vi "task_manager.vi"(8 "error out 2":errorcluster) -> (0 "error out":errorcluster)   [LabVIEW 2010]
uses:
  <userlib>/_OpenG.lib/array/array.llb/Sort 1D Array (String)__ogtk.vi
  <userlib>/_OpenG.lib/array/array.llb/Sort 2D Array (String)__ogtk.vi
panel:
  in  "sort by":u32(ring) items=["Name", "Type", "State", "Size", "Clones"]
  in  "stop":bool
  in  "end process":bool
  in  "VIs in Memory:":i32(listbox)
  # "Task Manager"
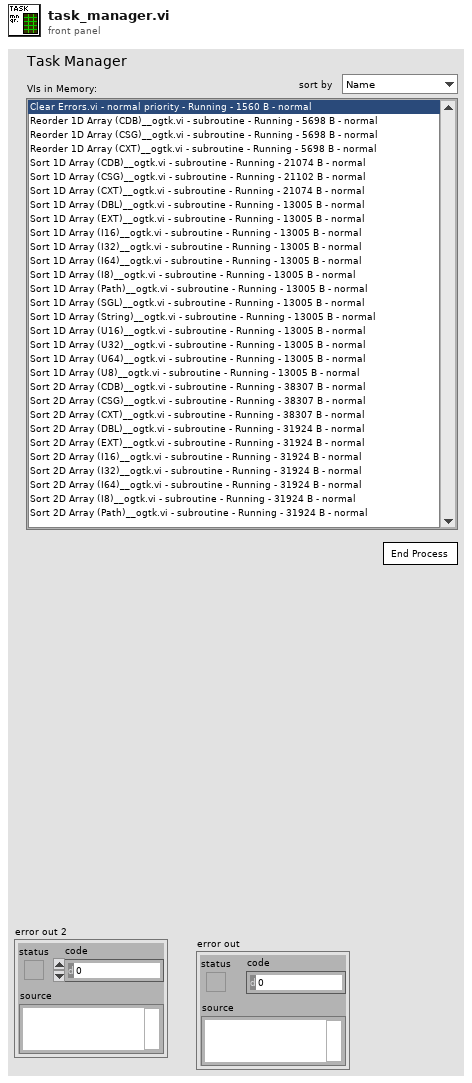
[diagram p1: front panel]
types:
  T1 = enum32{"invalid priority", "background priority", "normal priority", "above normal priority", "high priority", "time critical priority", "subroutine"}
  T2 = enum32{"Bad", "Idle", "Run top level", "Running"}
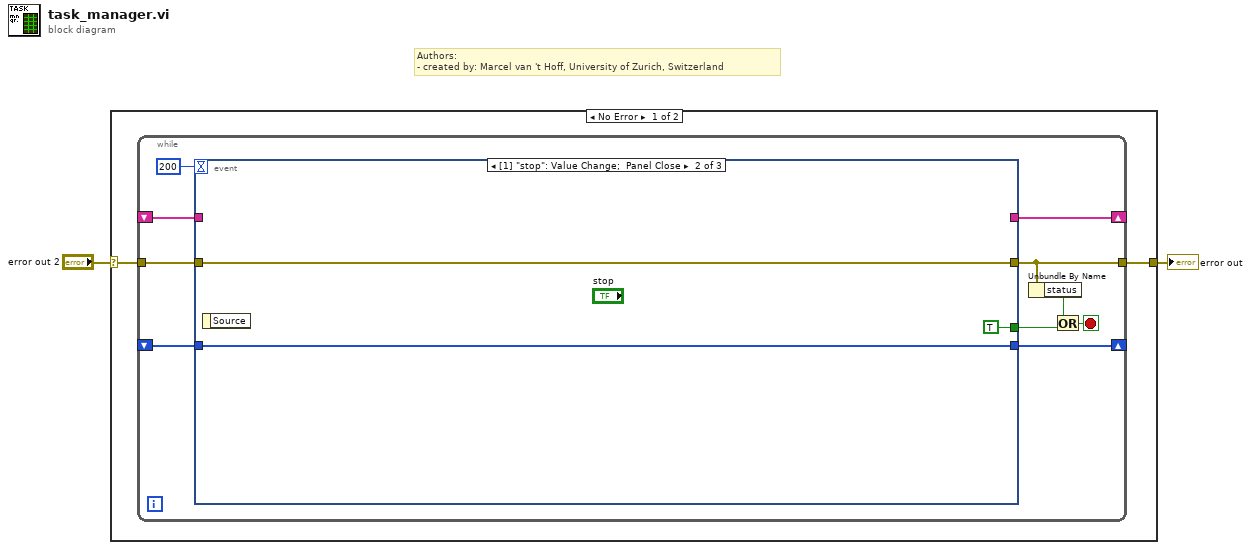
[diagram p0: block diagram]
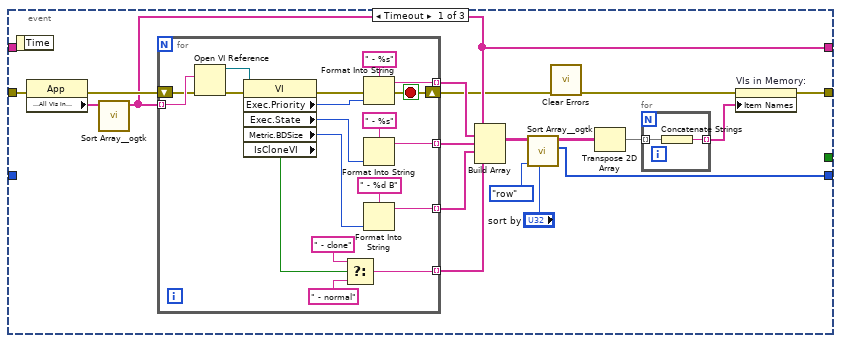
[diagram p2: hidden frame]
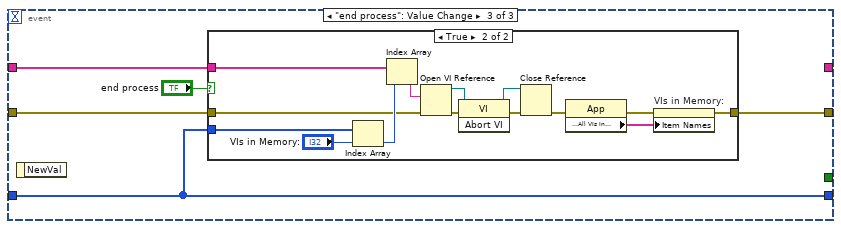
[diagram p3: hidden frame]
diagram:
  # "Authors: \n- created by: Marcel van 't Hoff, University of Zurich, Switzerland"
  n1 = case shown="No Error" "error out 2" {
    selector: "error out 2" -> [w3 w77]
    tunnel: [w4 w77] -> w2
    frame No Error {
      n2 = while {
        shift-right: [w13] -> _
        shift-left: _ -> [w12]
        shift-right: [w11] -> _
        shift-left: _ -> [w10]
        tunnel: [w8] -> w4
        tunnel: w3 -> [w9]
        stop <- w5 stop-if-true
        n3 = event shown="[1] \"stop\": Value Change;  Panel Close" {
          selector: _ -> [_ _ _]
          dyn-events: _ -> [_ _ _]
          timeout: 200 -> [_ _ _]
          tunnel: [_ TRUE ("stop") _] -> w6
          tunnel: [w18 _ _] -> w13
          tunnel: w12 -> [_ _ w60]
          tunnel: [w22 w56 w59] -> w11
          tunnel: w10 -> [_ w56 w59]
          tunnel: [w20 w55 w58] -> w8
          tunnel: w9 -> [w21 w55 w57]
          event Timeout {
            n4 = event-data() -> ()  [unwired: 1 in, 1 out]
            n5 = property class="App"(error in=w21) -> (error out=w19:errorcluster, "Application:All VIs In Memory"=w23:string[])  [unwired: 1 in, 1 out]
            n6 = call-poly <userlib>:"Sort Array__ogtk.vi"("Array in"=w23) -> ("Sorted Array out"=w18:string[])  [unwired: 9 in, 1 out]
            n7 = for {
              tunnel: w18 -> [w52] mode=indexing
              tunnel: [w46] -> w32 mode=indexing
              tunnel: [w45] -> w30 mode=indexing
              tunnel: [w44] -> w29 mode=indexing
              shift-right: [w39] -> w17
              shift-left: w19 -> [w41]
              tunnel: [w37] -> w16 mode=indexing
              stop <- w39 stop-if-true
              n8 = Open VI Reference(vi path=w52, error in (no error)=w41) -> (vi reference=w53:refnum<vi>, error out=w42:errorcluster)  [unwired: 4 in]
              n9 = property class="VI"(reference=w53, error in=w42) -> (error out=w40:errorcluster, "Exec.Priority"=w50:T1, "Exec.State"=w47:T2, "Metric.BDSize"=w43:u32, "IsCloneVI"=w38:bool)  [unwired: 1 out]
              n10 = Select(t=" - clone" ("format string"), s=w38, f=" - normal" ("format string")) -> (s? t:f=w37:string)
              n11 = Format Into String(format string=" - %s", error in=w40, w50) -> (resulting string=w46:string, error out=w39:errorcluster)  [unwired: 1 in]
              n12 = Format Into String(format string=" - %s", w47) -> (resulting string=w45:string)  [unwired: 2 in, 1 out]
              n13 = Format Into String(format string=" - %d B", w43) -> (resulting string=w44:string)  [unwired: 2 in, 1 out]
            }
            n14 = Build Array(w18, w32, w30, w29, w16) -> (w31:string[][])
            n15 = call-poly <userlib>:"Sort Array__ogtk.vi"("Column/Row to Sort By"="sort by", "Sort By in"=enum16{"row", "column"}."row", "Array in"=w31) -> ("Sorted Pointers"=w22:i32[], "Sorted Array out"=w28:string[][])  [unwired: 5 in, 2 out]
            n16 = call <vilib>:"Clear Errors.vi"("error in (no error)"=w17) -> ("error out"=w15:errorcluster)  [unwired: 6 in]
            n17 = Transpose 2D Array(2D array=w28) -> (transposed array=w26:string[][])
            n18 = for {
              tunnel: w26 -> [w34] mode=indexing
              tunnel: [w33] -> w27 mode=indexing
              n19 = Concatenate Strings(w34) -> (w33:string)
            }
            n20 = property on="VIs in Memory:" class="LstBox (strict)"(error in=w15, "Item Names"=w27) -> (error out=w20:errorcluster)  [unwired: 1 in, 1 out]
          }
          event "stop": Value Change; Panel Close {
            n21 = event-data() -> ()  [unwired: 1 in, 1 out]
          }
          event "end process": Value Change {
            n22 = event-data() -> ()  [unwired: 1 in, 1 out]
            n23 = case shown="True" "end process" {
              tunnel: w60 -> [_ w75]
              tunnel: w59 -> [_ w74]
              tunnel: [w62 w64] -> w58
              tunnel: w57 -> [w62 w63]
              frame False {
              }
              frame True {
                n24 = Index Array(array=w74, index="VIs in Memory:") -> (element=w72:i32)
                n25 = Index Array(array=w75, index=w72) -> (element=w76:string)
                n26 = Open VI Reference(vi path=w76, error in (no error)=w63) -> (vi reference=w71:refnum<vi>, error out=w70:errorcluster)  [unwired: 4 in]
                n27 = invoke class="VI" method="Abort VI"(reference=w71, error in=w70) -> (reference out=w69:refnum<vi>, error out=w68:errorcluster)  [unwired: 1 in, 1 out]
                n28 = Close Reference(reference=w69, error in (no error)=w68) -> (error out=w67:errorcluster)
                n29 = property class="App"(error in=w67) -> (error out=w65:errorcluster, "Application:All VIs In Memory"=w66:string[])  [unwired: 1 in, 1 out]
                n30 = property on="VIs in Memory:" class="LstBox (strict)"(error in=w65, "Item Names"=w66) -> (error out=w64:errorcluster)  [unwired: 1 in, 1 out]
              }
            }
          }
        }
        n31 = Unbundle By Name(w8) -> ("status"=w7:bool)
        n32 = Or(x=w7, y=w6) -> (x .or. y?=w5:bool)
      }
    }
    frame Error {
    }
  }
  "error out" <- w2
